vi "Connect to python.vi"() -> ()   [LabVIEW 2020]
uses:
  <vilib>/addons/zeromq/socket_type.ctl
  <vilib>/addons/zeromq/zmq_context.lvclass
  <vilib>/addons/zeromq/zmq_socket.lvclass
  <vilib>/addons/zeromq/zeromq.lvlib
panel:
  out "data":string
  in  "Numeric":i32=10
  out "Intensity Graph":dbl[][](graph)
  in  "Send req":bool
  in  "stop":bool
  in  "In":string="giveImage"
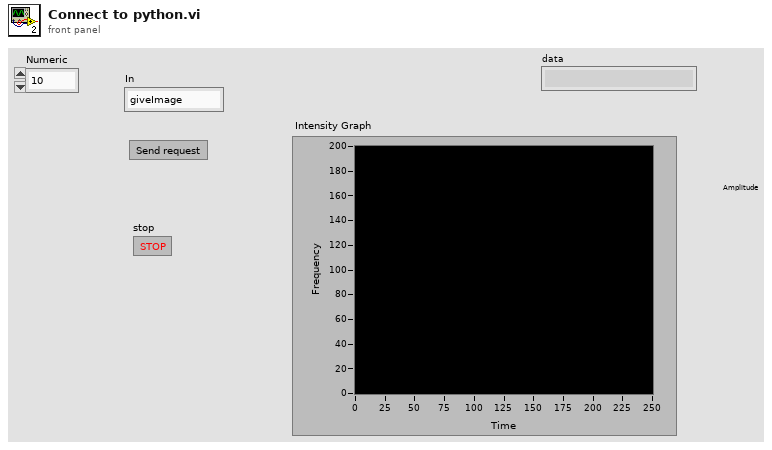
[diagram p1: front panel]
types:
  T1 = typedef "zeromq.lvlib/socket_type.ctl" = enum8{"ZMQ_PAIR", "ZMQ_PUB", "ZMQ_SUB", "ZMQ_REQ", "ZMQ_REP", "ZMQ_DEALER", "ZMQ_ROUTER", "ZMQ_PULL", "ZMQ_PUSH", "ZMQ_XPUB", "ZMQ_XSUB"}
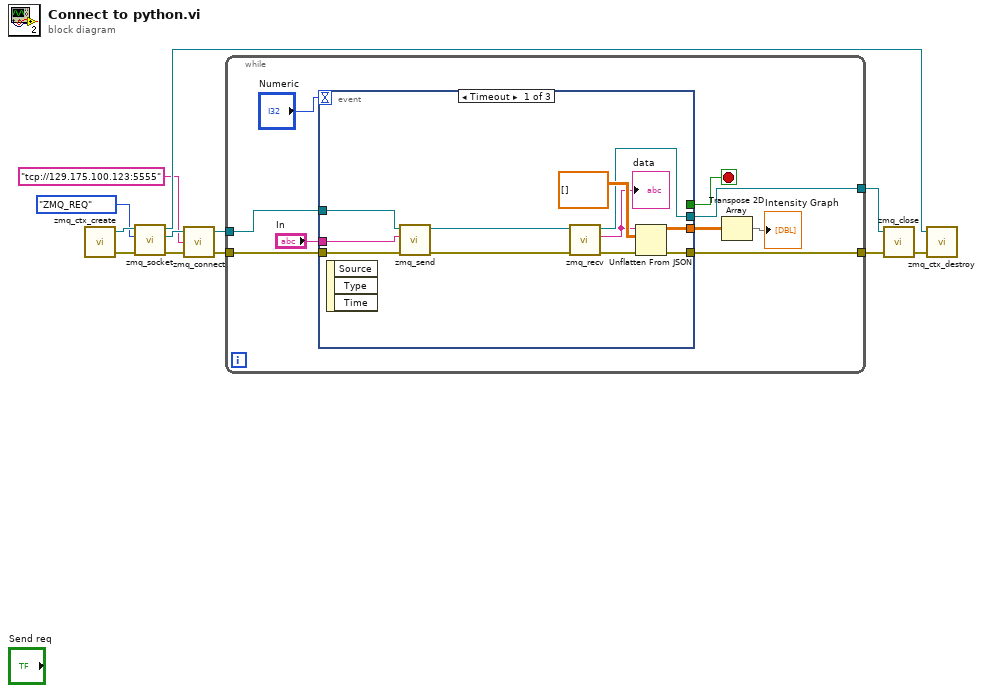
[diagram p0: block diagram]
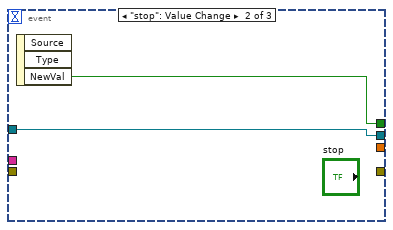
[diagram p2: hidden frame]
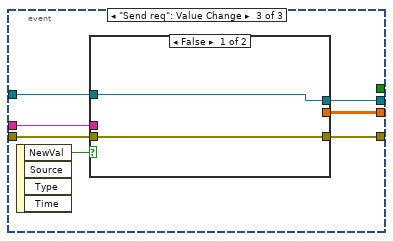
[diagram p3: hidden frame]
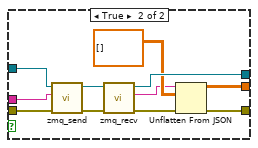
[diagram p4: hidden frame]
diagram:
  n1 = call <vilib>:"zmq_ctx_create.vi"() -> ("error out"=w11:errorcluster, "context out"=w12:refnum<class "zmq_context.lvclass">)  [unwired: 4 in]
  n2 = call <vilib>:"zmq_socket.vi"("error in"=w11, "socket type"=socket_type."ZMQ_REQ", "context in"=w12) -> ("error out"=w10:errorcluster, "socket out"=w7:refnum<class "zmq_socket.lvclass">, "context out"=w8:refnum<class "zmq_context.lvclass">)  [unwired: 2 in]
  n3 = call <vilib>:"zmq_connect.vi"("error in"=w10, "endpoint"="tcp://129.175.100.123:5555", "socket in"=w7) -> ("error out"=w3:errorcluster, "socket out"=w4:refnum<class "zmq_socket.lvclass">)  [unwired: 1 in]
  n4 = while {
    tunnel: w4 -> [w21]
    tunnel: w3 -> [w20]
    tunnel: [w17] -> w2
    tunnel: [w19] -> w1
    stop <- w18 stop-if-true
    n5 = event shown="[0] Timeout" {
      selector: _ -> [_ _ _]
      dyn-events: _ -> [_ _ _]
      timeout: "Numeric" -> [_ _ _]
      tunnel: w21 -> [w32 w33 w41]
      tunnel: w20 -> [w31 _ w40]
      tunnel: [w24 w33 w39] -> w19
      tunnel: [_ w34 _] -> w18
      tunnel: [w23 _ w38] -> w17
      tunnel: [w22 _ w36] -> w16
      tunnel: "In" -> [w25 _ w35]
      event Timeout {
        n6 = event-data() -> ()  [unwired: 1 in, 3 out]
        n7 = call <vilib>:"zmq_send.vi"("error in"=w31, "data"=w25, "socket in"=w32) -> ("error out"=w30:errorcluster, "socket out"=w29:refnum<class "zmq_socket.lvclass">)  [unwired: 4 in]
        n8 = call <vilib>:"zmq_recv.vi"("error in"=w30, "socket in"=w29) -> ("error out"=w27:errorcluster, "data"=w26:string, "socket out"=w24:refnum<class "zmq_socket.lvclass">)  [unwired: 3 in, 2 out]
        "data" <- w26
        n9 = Unflatten From JSON(JSON string=w26, type and defaults=dbl[][] [] ("array"), error in (no error)=w27) -> (value=w22:dbl[][], error out=w23:errorcluster)  [unwired: 4 in]
      }
      event "stop": Value Change {
        n10 = event-data() -> ("NewVal"=w34:bool)  [unwired: 1 in, 2 out]
      }
      event "Send req": Value Change {
        n11 = event-data() -> ("NewVal"=w37:bool)  [unwired: 1 in, 3 out]
        n12 = case shown="False" w37 {
          tunnel: w41 -> [w43 w52]
          tunnel: w40 -> [w42 w51]
          tunnel: [w43 w50] -> w39
          tunnel: [w42 w48] -> w38
          tunnel: [_ w45] -> w36
          tunnel: w35 -> [_ w44]
          frame False {
          }
          frame True {
            n13 = call <vilib>:"zmq_send.vi"("error in"=w51, "data"=w44, "socket in"=w52) -> ("error out"=w54:errorcluster, "socket out"=w53:refnum<class "zmq_socket.lvclass">)  [unwired: 4 in]
            n14 = call <vilib>:"zmq_recv.vi"("error in"=w54, "socket in"=w53) -> ("error out"=w47:errorcluster, "data"=w46:string, "socket out"=w50:refnum<class "zmq_socket.lvclass">)  [unwired: 3 in, 2 out]
            n15 = Unflatten From JSON(JSON string=w46, type and defaults=dbl[][] [] ("array"), error in (no error)=w47) -> (value=w45:dbl[][], error out=w48:errorcluster)  [unwired: 4 in]
          }
        }
      }
    }
    n16 = Transpose 2D Array(2D array=w16) -> (transposed array=→"Intensity Graph":dbl[][])
  }
  n17 = call <vilib>:"zmq_close.vi"("error in"=w2, "socket"=w1) -> ("error out"=w9:errorcluster)  [unwired: 3 in]
  n18 = call <vilib>:"zmq_ctx_destroy.vi"("error in"=w9, "context in"=w8) -> ()  [unwired: 3 in, 1 out]
